vi "Agilent PWM Wait for Operation Complete (OPC).vi"(8 "error in (no error)":errorcluster, 10 "Timeout, ms (10000)":u32=10000, 11 "VISA Resource Name":refnum<visa-resource-name>) -> (0 "error out":errorcluster, 3 "dup VISA Resource Name":refnum<visa-resource-name>)   [LabVIEW 2011]
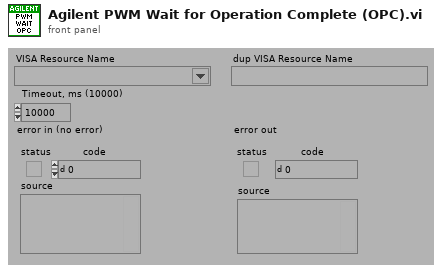
[diagram p1: front panel]
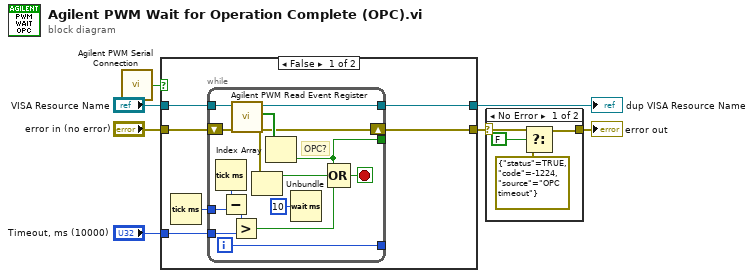
[diagram p0: block diagram]
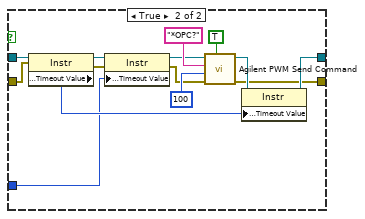
[diagram p2: hidden frame]
diagram:
  n1 = call "Agilent PWM Serial Connection.vi"("VISA Resource Name"="VISA Resource Name") -> ("Serial?"=w6:bool)
  n2 = case shown="False" w6 {
    tunnel: [w11 w29] -> w2
    tunnel: "Timeout, ms (10000)" -> [w8 w38]
    tunnel: "error in (no error)" -> [w13 w39]
    tunnel: "VISA Resource Name" -> [w12 w36]
    tunnel: [w10 w37] -> w1
    frame False {
      n3 = Tick Count (ms)() -> (millisecond timer value=w9:u32)
      n4 = while {
        tunnel: [w19] -> _
        tunnel: w12 -> [w23]
        tunnel: w8 -> [w25]
        tunnel: w9 -> [w28]
        shift-right: [w20] -> w11
        shift-left: w13 -> [w21]
        tunnel: [w15] -> w10
        tunnel: [w14] -> _
        i -> [w14]
        stop <- w16 stop-if-true
        # "OPC?"
        n5 = Tick Count (ms)() -> (millisecond timer value=w27:u32)
        n6 = Subtract(x=w27, y=w28) -> (x-y=w26:u32)
        n7 = Greater?(x=w26, y=w25) -> (0:w17:bool)
        n8 = call "Agilent PWM Read Event Register.vi"("error in (no error)"=w21, "VISA Resource Name"=w23) -> ("error out"=w20:errorcluster, "Event Register"=w22:bool[], "dup VISA Resource Name"=w15:refnum<visa-resource-name>)  [unwired: 7 out]
        n9 = Unbundle(w20) -> ("status"=w18:bool)  [unwired: 2 out]
        n10 = Index Array(array=w22) -> (element=w19:bool)  [unwired: 1 in]
        n11 = Wait (ms)(milliseconds to wait=u32 10) -> ()  [unwired: 1 out]
        n12 = Compound Arithmetic op=OR(w19, w18, w17) -> (w16:bool)
      }
    }
    frame True {
      n13 = property on="Property Node" class="Instr"(reference=w36, error in=w39) -> (reference out=w42:refnum<visa-resource-name>, error out=w41:errorcluster, "General Settings:Timeout Value"=w40:u32)
      n14 = property on="Property Node" class="Instr"(reference=w42, error in=w41, "General Settings:Timeout Value"=w38) -> (reference out=w31:refnum<visa-resource-name>, error out=w32:errorcluster)
      n15 = call "Agilent PWM Send Command.vi"("Read? (F)"=TRUE ("use system decimal point (T)"), "error in (no error)"=w32, "Byte Count"=u32 100, "Command"="*OPC?", "VISA Resource Name"=w31) -> ("error out"=w29:errorcluster, "dup VISA Resource Name"=w30:refnum<visa-resource-name>)  [unwired: 5 out]
      n16 = property on="Property Node" class="Instr"(reference=w30, "General Settings:Timeout Value"=w40) -> (reference out=w37:refnum<visa-resource-name>)  [unwired: 1 in, 1 out]
    }
  }
  "dup VISA Resource Name" <- w1
  n17 = case shown="No Error" w2 {
    selector: w2 -> [w46 w47]
    tunnel: [w45 w47] -> w7
    frame No Error {
      n18 = Select(t=w46, s=FALSE, f=errorcluster {"status"=TRUE, "code"=-1224, "source"="OPC timeout"}) -> (s? t:f=w45:errorcluster)
    }
    frame Error {
    }
  }
  "error out" <- w7
